vi "DSF.Engine.BuilderManager.Build.vi"(8 "error in (no error)":errorcluster, 11 "Builder Manager in":refnum<class "DSF.Engine.BuilderManager.lvclass">) -> (0 "error out":errorcluster, 3 "Builder Manager out":refnum<class "DSF.Engine.BuilderManager.lvclass">)   [LabVIEW 2016, in "DSF.Engine.lvlib" / "DSF.Engine.BuilderManager.lvclass"]
uses:
  DSF.Engine.BuilderManager.lvclass
  Builder/DSF.Engine.Builder.lvclass
  Interface/DSF.Engine.Interface.Builder.lvclass
  Interface/DSF.Engine.Interface.Builder.Write.Command.vi
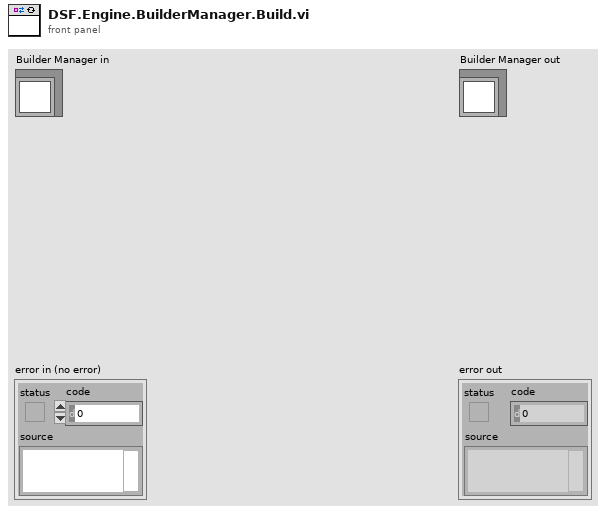
[diagram p1: front panel]
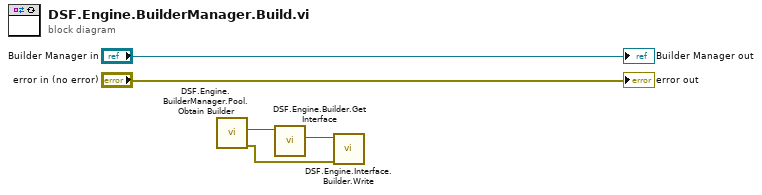
[diagram p0: block diagram]
diagram:
  n1 = call "DSF.Engine.BuilderManager.Pool.Obtain Builder.vi"() -> ("error out"=w1:errorcluster, "Builder"=w3:refnum<class "DSF.Engine.Builder.lvclass">)  [unwired: 9 in, 1 out]
  n2 = call "DSF.Engine.Builder.Get Interface.vi"("Builder in"=w3) -> ("Builder Interface"=w2:refnum<class "DSF.Engine.Interface.Builder.lvclass">)  [unwired: 9 in, 1 out]
  n3 = call-poly "DSF.Engine.Interface.Builder.Write.vi"("error in (no error)"=w1, "Builder Interface in"=w2) -> ()  [unwired: 7 in, 3 out]
  "error out" <- "error in (no error)"
  "Builder Manager out" <- "Builder Manager in"
